vi "dual_channel_spectral.vi"(0 "Input Signal A":dynamicdata(graph), 2 "Input Signal B":dynamicdata(graph), 3 "Restart Averaging (F)":bool, 5 "error in (no error)":errorcluster, 8 "Averaging parameters":T2={"averaging mode"=enum."Vector averaging", "weighting mode"=enum."Exponential", "number of averages"=10}, 10 "Window":T1(ring)=enum."Hanning", 11 "unwrap phase (F)":bool) -> (9 "Averaging Done":bool, 14 "Magnitude":dynamicdata(graph), 16 "Phase":dynamicdata(graph), 17 "Imaginary":dynamicdata(graph), 18 "Real":dynamicdata(graph), 19 "error out":errorcluster)   [LabVIEW 2013]
doc: "Performs the dual channel spectral measurement of the frequency repsonse function on a signal.\n--------------------\n\nThis Express VI is configured as follows:\n\nSelected Measurements: Power Spectal Density\nMagnitude, Phase, View Phase: Wrapped and in Radians\nWindowing: Blackman\nAveraging: None"
panel:
  in  "Tab Control":T3(tab)
  out "Coherence":dynamicdata(graph)
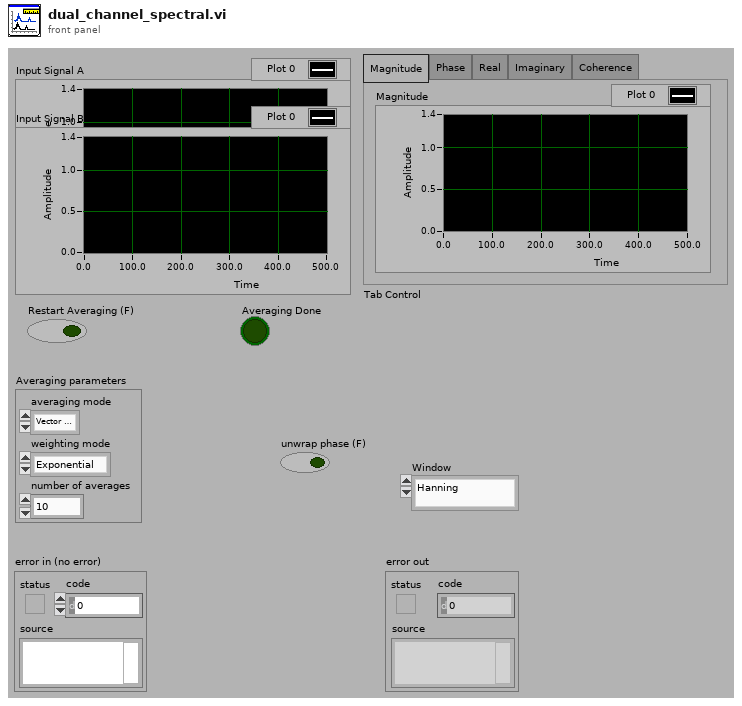
[diagram p1: front panel]
types:
  T1 = enum16{"None ", "Hanning", "Hamming", "Blackman-Harris", "Exact Blackman", "Blackman", "Flat Top", "4 Term B-Harris ", "7 Term B-Harris", "Low Sidelobe"}
  T2 = cluster{"averaging mode":enum16{"No averaging", "Vector averaging", "RMS averaging", "Peak hold"}, "weighting mode":enum16{"Linear", "Exponential"}, "number of averages":u32}
  T3 = enum32{"Magnitude", "Phase", "Real", "Imaginary", "Coherence"}
  T4 = cluster{"dB On (F)":bool, "unwrap phase (F)":bool, "convert to degree (F)":bool}
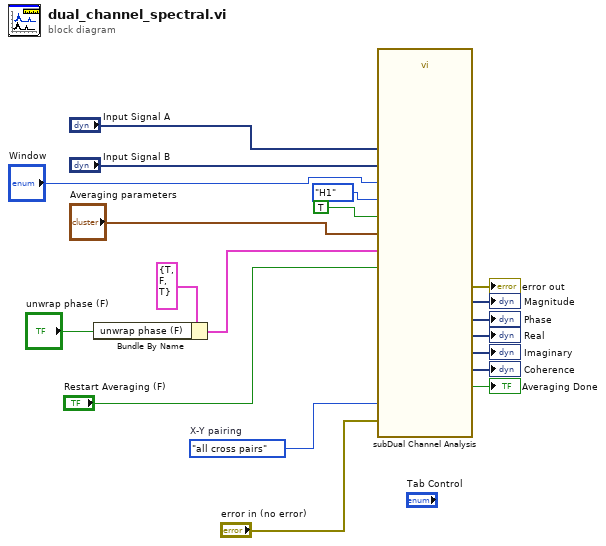
[diagram p0: block diagram]
diagram:
  w6 = enum32{"ordered pairs", "all cross pairs"}."all cross pairs"  # X-Y pairing
  n1 = Bundle By Name(cluster=T4 {"dB On (F)"=TRUE, "unwrap phase (F)"=FALSE, "convert to degree (F)"=TRUE} ("view"), "unwrap phase (F)"="unwrap phase (F)") -> (w3:T4)
  n2 = call <vilib>:"subDual Channel Analysis.vi"("Input Signal A"="Input Signal A", "Input Signal B"="Input Signal B", "X-Y pairing"=w6, "Restart Averaging (F)"="Restart Averaging (F)", "Window"="Window", "error in (no error)"="error in (no error)", "view"=w3, "averaging parameters"="Averaging parameters", "FRF Mode"=enum16{"H1", "H2", "H3"}."H1", "Every iteration"=TRUE) -> ("Magnitude"=→"Magnitude":dynamicdata, "Averaging Done"=→"Averaging Done":bool, "Phase"=→"Phase":dynamicdata, "Real"=→"Real":dynamicdata, "Imaginary"=→"Imaginary":dynamicdata, "Coherence"=→"Coherence":dynamicdata, "error out"=→"error out":errorcluster)  [unwired: 3 out]
